vi "Open RIO Camera.vi"(8 "error in (no error)":errorcluster, 10 "Remote Host":string="roborio-836-frc.local", 11 "Port":u16=5800) -> (0 "error out":errorcluster, 3 "Cluster":T1)   [LabVIEW 2015]
uses:
  Camera Network Settings.ctl
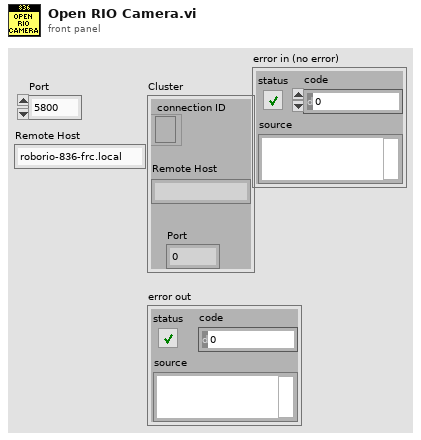
[diagram p1: front panel]
types:
  T1 = typedef "Camera Network Settings.ctl" = cluster{"connection ID":refnum<k5>, "Port":u16, "Remote Host":string}
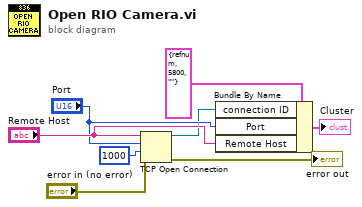
[diagram p0: block diagram]
diagram:
  n1 = TCP Open Connection(address="Remote Host", remote port or service name="Port", timeout ms (60000)=1000, error in (no error)="error in (no error)") -> (connection ID=w5:refnum<k5>, error out=→"error out":errorcluster)  [unwired: 1 in]
  n2 = Bundle By Name(cluster=T1 {"connection ID"=refnum, "Port"=5800, "Remote Host"=""}, "connection ID"=w5, "Port"="Port", "Remote Host"="Remote Host") -> (→"Cluster":T1)
